vi "Incorrect EtherCAT Variable 6203--error.vi"() -> (0 "error out":errorcluster)   [LabVIEW 2024, in "EtherCAT Model.lvlib"]
uses:
  EtherCAT Model.lvlib
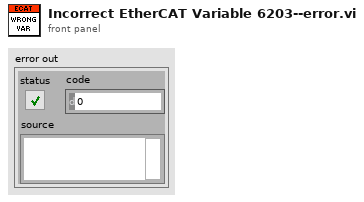
[diagram p1: front panel]
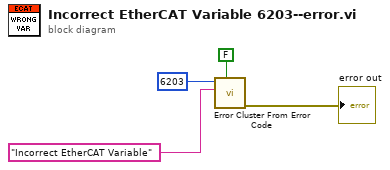
[diagram p0: block diagram]
diagram:
  n1 = call <vilib>:"Error Cluster From Error Code.vi"("show call chain? (False)"=FALSE, "error message (\"\")"="Incorrect EtherCAT Variable" ("error message (\"\")"), "error code (0)"=6203) -> ("error out"=→"error out":errorcluster)  [unwired: 6 in]
